vi "CloseHS.vi"(8 "error in (no error)":errorcluster, 11 "Python":T1) -> ()   [LabVIEW 2024]
uses:
  PythonCtrl.ctl
  Processors.ctl
panel:
  out "return value":string
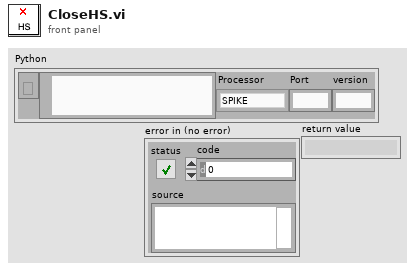
[diagram p1: front panel]
types:
  T1 = typedef "PythonCtrl.ctl" = cluster{"session":refnum<k35>, "PyPath":path, "Processor":T2, "Port":string, "version":string}
  T2 = typedef "Processors.ctl" = enum16{"SPIKE", "Pi", "Pi_ssh", "OpenMV", "Dunio"}
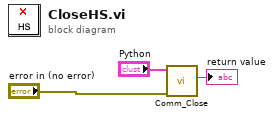
[diagram p0: block diagram]
diagram:
  n1 = call "Comm_Close.vi"("error in (no error)"="error in (no error)", "Python in"="Python") -> ("return value"=→"return value":string)  [unwired: 8 in, 1 out]
